vi "rethinkdb_example_query.vi"() -> ()   [LabVIEW 2017]
uses:
  rethinkdb/msg/rethinkdb_msg_connect_auth.ctl
  rethinkdb/json/json_element_type.ctl
  rethinkdb/ast/ast_db.vi
  rethinkdb/ast/ast_db_list.vi
  rethinkdb/ast/ast_reql_cache.vi
  <vilib>/Utility/error.llb/Error Cluster From Error Code.vi
  rethinkdb/rethinkdb.lvclass
panel:
  in  "elements":T2(array[cluster])
  out "response":string
  in  "auth":T3={"user"="ryan", "password"="ryan"}
  in  "host (\"localhost\")":string="localhost"
  in  "port (28015)":u16=28015
  in  "ms timeout (10000)":i32=10000
  out "error out":errorcluster
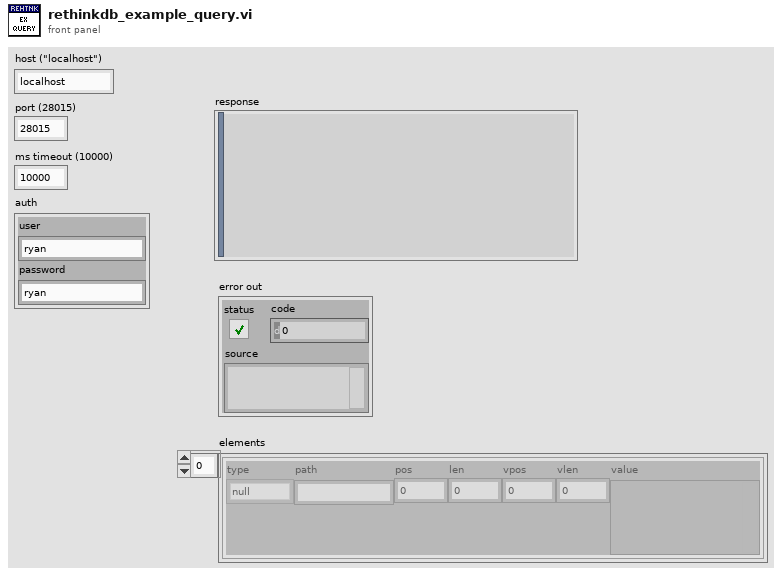
[diagram p1: front panel]
types:
  T1 = typedef "json_element_type.ctl" = enum8{"null", "bool", "int", "uint", "float", "string", "array", "object"}
  T2 = cluster{"type":T1, "path":string, "pos":i32, "len":i32, "vpos":i32, "vlen":i32, "value":variant}[]
  T3 = typedef "rethinkdb_msg_connect_auth.ctl" = cluster{"user":string, "password":string}
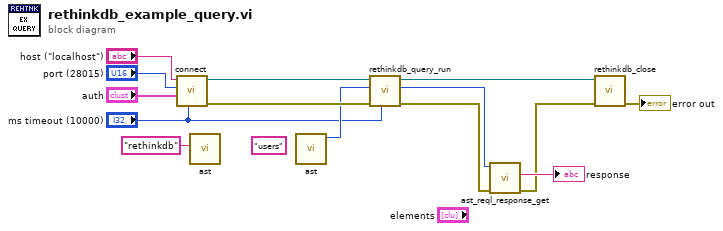
[diagram p0: block diagram]
diagram:
  (unwired) "users" ("table_name")
  n1 = call "connect.vi"("ms timeout (10000)"="ms timeout (10000)", "auth"="auth", "port (28015)"="port (28015)", "host (\"localhost\")"="host (\"localhost\")") -> ("error out"=w7:errorcluster, "rethinkdb"=w6:refnum<k5>)  [unwired: 5 in, 1 out]
  n2 = call-poly "ast.vi"("db_name"="rethinkdb") -> ()  [unwired: 10 in, 1 out]
  n3 = call-poly "ast.vi"() -> ("rql_query"=w5:u32)  [unwired: 11 in]
  n4 = call "rethinkdb_query_run.vi"("timeout ms (10000)"="ms timeout (10000)", "error in (no error)"=w7, "reql_id in"=w5, "rethinkdb in"=w6) -> ("error out"=w3:errorcluster, "reql_id out"=w2:u32, "rethinkdb out"=w1:refnum<k5>)  [unwired: 5 in]
  n5 = call "ast_reql_response_get.vi"("error in (no error)"=w3, "reql_id in"=w2) -> ("error out"=w8:errorcluster, "response"=→"response":string)  [unwired: 7 in, 1 out]
  n6 = call "rethinkdb_close.vi"("error in (no error)"=w8, "rethinkdb in"=w1) -> ("error out"=→"error out":errorcluster)  [unwired: 9 in]
